vi "G#Object_ByteArrayToVariant.vi"(2 "unsigned byte array":u8[](array[numeric]), 5 "error in":errorcluster, 6 "type string":i16[](array[numeric])) -> (15 "variant":variant, 19 "error out":errorcluster)   [LabVIEW 2017, in "G#Object.lvclass"]
uses:
  G#Object.lvclass
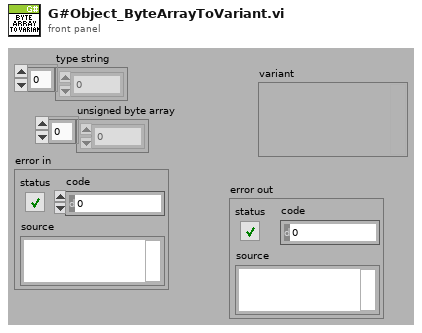
[diagram p1: front panel]
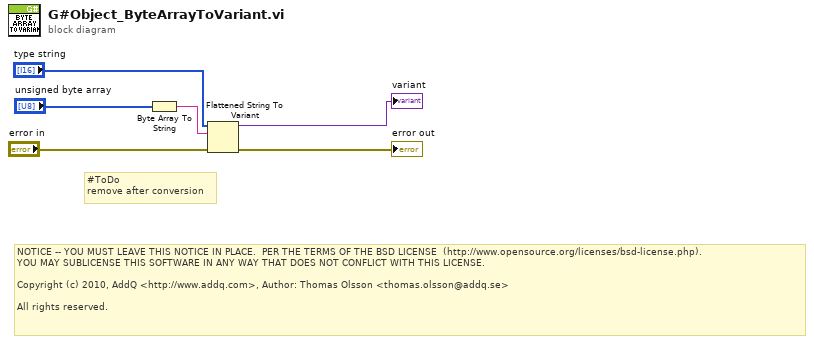
[diagram p0: block diagram]
diagram:
  # "#ToDo\nremove after conversion"
  # "NOTICE -- YOU MUST LEAVE THIS NOTICE IN PLACE.  PER THE TERMS OF THE BSD LICENSE  (http://www.opensource.org/licenses/bsd-license.php).\nYOU MAY SUBLICENSE THIS SOFTWARE IN ANY WAY THAT DOES NOT CONFLICT WITH THIS LICENSE.\n\nCopyright (c) 2010, AddQ <http://www.addq.com>, Author: Thomas Olsson <thomas.olsson@addq.se>\n\nAll rights reserved."
  n1 = Byte Array To String(unsigned byte array="unsigned byte array") -> (string=w6:string)
  n2 = Flattened String To Variant(4:"error in", 6:w6, 7:"type string") -> (0:→"error out":errorcluster, 3:→"variant":variant)
